vi "Set NULL.vi"(10 "NULL":bool, 11 "Type in":refnum<class "Type.lvclass">) -> (3 "Type out":refnum<class "Type.lvclass">)   [LabVIEW 2022 SP3, in "Conditum.lvlib" / "Columns.lvlib" / "Type.lvclass"]
uses:
  Type.lvclass
  Type.lvclass/Type.ctl
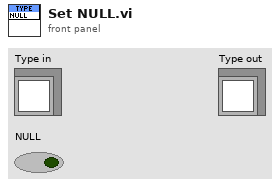
[diagram p1: front panel]
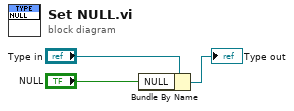
[diagram p0: block diagram]
diagram:
  n1 = Bundle By Name(cluster="Type in", "NULL"="NULL") -> (→"Type out":refnum<class "Type.lvclass">)
